vi "Run BAT.vi"(7 "working directory":path=path "C:/Users/omartinez/Desktop", 8 "error in":errorcluster, 11 "filename":string="test.bat") -> (0 "error out":errorcluster)   [LabVIEW 2012]
panel:
  out "standard output":string
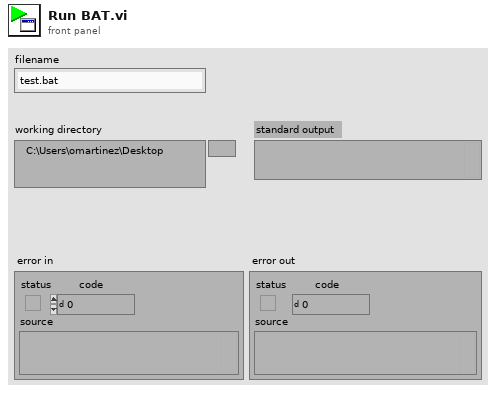
[diagram p1: front panel]
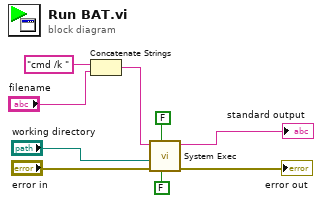
[diagram p0: block diagram]
diagram:
  n1 = Concatenate Strings("cmd /k " ("command line"), "filename") -> (w2:string)
  n2 = call <vilib>:"System Exec.vi"("run minimized? (F)"=FALSE, "wait until completion? (T)"=FALSE, "error in (no error)"="error in", "working directory"="working directory", "command line"=w2) -> ("error out"=→"error out":errorcluster, "standard output"=→"standard output":string)  [unwired: 3 in, 2 out]
